vi "Update Recurrences.vi"(2 "Iterations (1)":i32=1, 3 "ExpenseMap":map{string, refnum<class "ATransfer.lvclass">}(c390), 4 "AccountMap":T1(c390)) -> (0 "ExpenseMap out":map{string, refnum<class "ATransfer.lvclass">}(c390), 1 "AccountMap out":T1(c390))   [LabVIEW 2020]
uses:
  Shared/IInterest/IInterest.lvclass
  shared/IAccountable/IAccountable.lvclass
  Shared/ATransfer/ATransfer.lvclass
  shared/IBasicAccount/IBasicAccount.lvclass
  C:/projects/budget_LabVIEW/Main Codeline/Software/Code/shared/IBasicAccount/IBasicAccount.lvclass
  C:/projects/budget_LabVIEW/Main Codeline/Software/Code/Shared/IDepositable/IDepositable.lvclass
  C:/projects/budget_LabVIEW/Main Codeline/Software/Code/Shared/IWithdrawable/IWithdrawable.lvclass
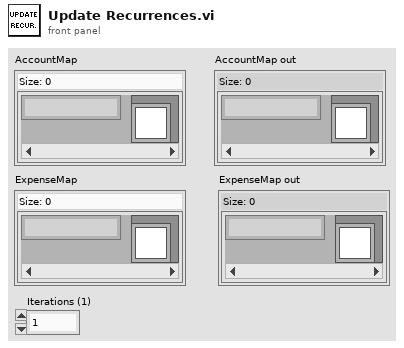
[diagram p1: front panel]
types:
  T1 = map{string, refnum<class "IBasicAccount.lvclass">}
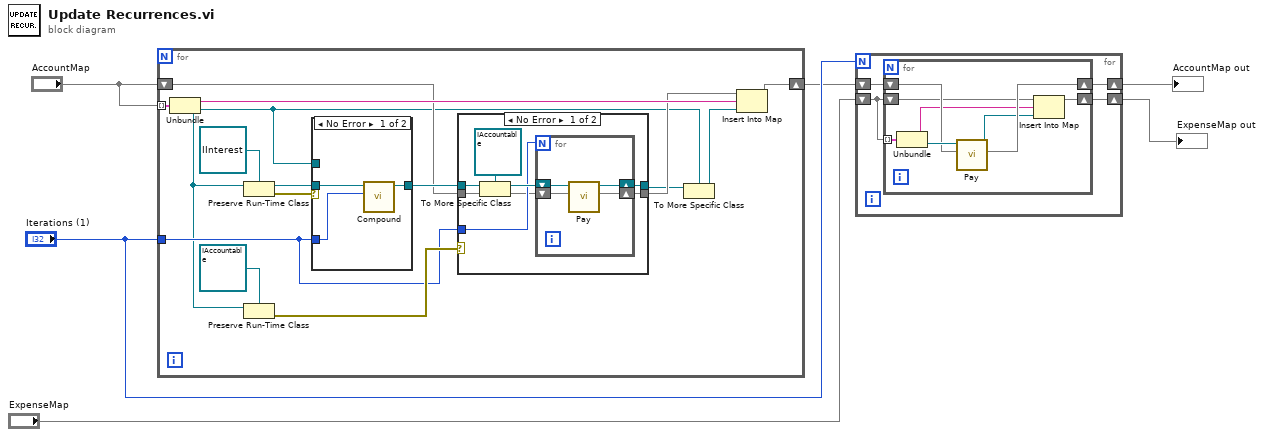
[diagram p0: block diagram]
diagram:
  n1 = for {
    shift-right: [w21] -> w4
    shift-left: "AccountMap" -> [w11]
    tunnel: "AccountMap" -> [w20] mode=indexing
    tunnel: "Iterations (1)" -> [w12]
    n2 = Unbundle(w20) -> (w19:string, "IBasicAccount.lvclass"=w8:refnum<class "IBasicAccount.lvclass">)
    n3 = Preserve Run-Time Class(object in=w8, 2:refnum<class "IInterest.lvclass"> refnum ("IInterest.lvclass")) -> (object out=w15:refnum<class "IInterest.lvclass">, error out=w16:errorcluster)  [unwired: 1 in]
    n4 = Preserve Run-Time Class(object in=w8, 2:refnum<class "IAccountable.lvclass"> refnum ("IAccountable.lvclass")) -> (error out=w14:errorcluster)  [unwired: 1 in, 1 out]
    n5 = case shown="No Error" w16 {
      tunnel: w15 -> [w37 _]
      tunnel: w12 -> [w36 _]
      tunnel: [w35 w38] -> w13
      tunnel: w8 -> [_ w38]
      frame No Error {
        n6 = call-dynamic "Compound.vi"("Timespan"=w36, "IInterest in"=w37) -> ("IInterest out"=w35:refnum<class "IInterest.lvclass">)  [unwired: 8 in, 1 out]
      }
      frame Error {
      }
    }
    n7 = case shown="No Error" w14 {
      tunnel: w13 -> [w28 w34]
      tunnel: w12 -> [w25 _]
      tunnel: w11 -> [w24 w33]
      tunnel: [w23 w33] -> w10
      tunnel: [w22 w34] -> w9
      frame No Error {
        n8 = To More Specific Class(target class=refnum<class "IAccountable.lvclass"> refnum ("IAccountable.lvclass"), reference=w28) -> (specific class reference=w26:refnum<class "IAccountable.lvclass">)  [unwired: 1 in, 1 out]
        n9 = for {
          N: w25 -> [_]
          shift-right: [w31] -> w22
          shift-left: w26 -> [w32]
          shift-right: [w29] -> w23
          shift-left: w24 -> [w30]
          n10 = call-dynamic "Pay.vi"("Accoounts"=w30, "IAccountable in"=w32) -> ("Accoounts out"=w29:T1, "IAccountable out"=w31:refnum<class "IAccountable.lvclass">)  [unwired: 7 in, 1 out]
        }
      }
      frame Error {
      }
    }
    n11 = To More Specific Class(target class=w8, reference=w9) -> (specific class reference=w7:refnum<class "IBasicAccount.lvclass">)  [unwired: 1 in, 1 out]
    n12 = Insert Into Map(map in=w10, key=w19, value=w7) -> (map out=w21:T1)  [unwired: 2 out]
  }
  n13 = for {
    N: "Iterations (1)" -> [_]
    shift-right: [w41] -> w2
    shift-left: w4 -> [w42]
    shift-right: [w39] -> w1
    shift-left: "ExpenseMap" -> [w40]
    n14 = for {
      tunnel: w40 -> [w50] mode=indexing
      shift-right: [w47] -> w41
      shift-left: w42 -> [w48]
      shift-right: [w43] -> w39
      shift-left: w40 -> [w46]
      n15 = Unbundle(w50) -> (w45:string, "ATransfer.lvclass"=w49:refnum<class "ATransfer.lvclass">)
      n16 = call-dynamic "Pay.vi"("Accoounts"=w48, "ATransfer in"=w49) -> ("Accoounts out"=w47:T1, "ATransfer out"=w44:refnum<class "ATransfer.lvclass">)  [unwired: 7 in, 1 out]
      n17 = Insert Into Map(map in=w46, key=w45, value=w44) -> (map out=w43:map{string, refnum<class "ATransfer.lvclass">})  [unwired: 2 out]
    }
  }
  "AccountMap out" <- w2
  "ExpenseMap out" <- w1
